vi "ReadSizeMat_Image.vi"(8 "error in":errorcluster, 11 "Image Reference In":T1) -> (0 "error out":errorcluster, 1 "Height":i32, 2 "Width":i32, 3 "Image Reference Out":T1, 4 "Channel":i32)   [LabVIEW 2020, in "OpenLvVision_OpenCv.lvlib"]
doc: "Read size of the datatype\nNo malleable to breake vi inlining!"
uses:
  OpenLvVision_OpenCv.lvlib
  <vilib>/OpenLvVision/OpenLvVision_Image/Management/TypeDef/OLV Image.ctl
  <vilib>/OpenLvVision/OpenLvVision_Image/Management/OLV Management.lvlib
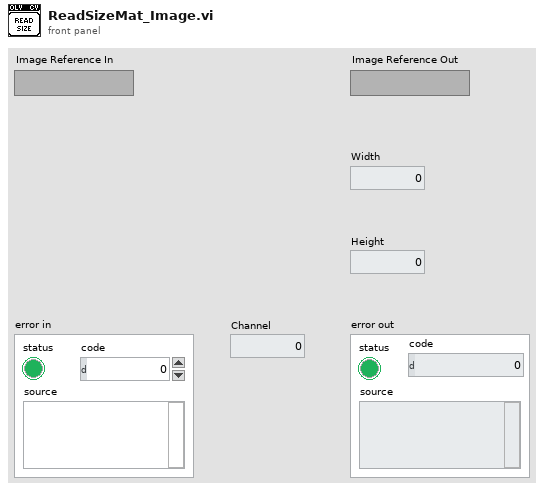
[diagram p1: front panel]
types:
  T1 = typedef "OLV OpenLvVision_Image.lvlib/OLV Management.lvlib/OLV Image.ctl" = refnum<image>
  T2 = typedef "OLV OpenLvVision_Image.lvlib/OLV Management.lvlib/OLV ImageType.ctl" = enum16{"Mono U8", "Mono U16", "Mono I16", "Mono SGL", "Color U32", "Color U64", "Complex CSG"}
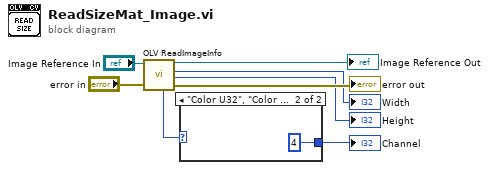
[diagram p0: block diagram]
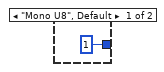
[diagram p2: hidden frame]
diagram:
  n1 = call <vilib>:"OLV ReadImageInfo.vi"("error in"="error in", "Image Reference In"="Image Reference In") -> ("error out"=→"error out":errorcluster, "Height"=→"Height":i32, "Width"=→"Width":i32, "Image Reference Out"=→"Image Reference Out":T1, "Image Type"=w8:T2)  [unwired: 4 in, 1 out]
  n2 = case shown="\"Color U32\", \"Color U64\"" w8 {
    tunnel: [1 4] -> w5
    frame "Mono U8", Default {
    }
    frame "Color U32", "Color U64" {
    }
  }
  "Channel" <- w5
